vi "Send 2 PC.vi"(8 "error in (no error)":errorcluster, 10 "port":u16=5800, 11 "Camera Data In":T1 {"Camera Settings"."VideoMode" items=["640 x 480 YUY 2 30.00 fps", "640 x 480 YUY 2 20.00 fps", "640 x 480 YUY 2 15.00 fps", "640 x 480 YUY 2 10.00 fps", "640 x 480 YUY 2 7.50 fps", "1280 x 720 YUY 2 10.00 fps", "1280 x 720 YUY 2 7.50 fps", "960 x 544 YUY 2 15.00 fps", "960 x 544 YUY 2 10.00 fps", "960 x 544 YUY 2 7.50 fps", "800 x 448 YUY 2 20.00 fps", "800 x 448 YUY 2 15.00 fps", "800 x 448 YUY 2 10.00 fps", "800 x 448 YUY 2 7.50 fps", "640 x 360 YUY 2 30.00 fps", "640 x 360 YUY 2 20.00 fps", "640 x 360 YUY 2 15.00 fps", "640 x 360 YUY 2 10.00 fps", "640 x 360 YUY 2 7.50 fps", "424 x 240 YUY 2 30.00 fps", "424 x 240 YUY 2 20.00 fps", "424 x 240 YUY 2 15.00 fps", "424 x 240 YUY 2 10.00 fps", "424 x 240 YUY 2 7.50 fps", "352 x 288 YUY 2 30.00 fps", "352 x 288 YUY 2 20.00 fps", "352 x 288 YUY 2 15.00 fps", "352 x 288 YUY 2 10.00 fps", "352 x 288 YUY 2 7.50 fps", "320 x 240 YUY 2 30.00 fps", "320 x 240 YUY 2 20.00 fps", "320 x 240 YUY 2 15.00 fps", "320 x 240 YUY 2 10.00 fps", "320 x 240 YUY 2 7.50 fps", "800 x 600 YUY 2 15.00 fps", "800 x 600 YUY 2 10.00 fps", "800 x 600 YUY 2 7.50 fps", "176 x 144 YUY 2 30.00 fps", "176 x 144 YUY 2 20.00 fps", "176 x 144 YUY 2 15.00 fps", "176 x 144 YUY 2 10.00 fps", "176 x 144 YUY 2 7.50 fps", "160 x 120 YUY 2 30.00 fps", "160 x 120 YUY 2 20.00 fps", "160 x 120 YUY 2 15.00 fps", "160 x 120 YUY 2 10.00 fps", "160 x 120 YUY 2 7.50 fps", "1280 x 800 YUY 2 10.00 fps", "640 x 480 JPEG 30.00 fps", "640 x 480 JPEG 20.00 fps", "640 x 480 JPEG 15.00 fps", "640 x 480 JPEG 10.00 fps", "640 x 480 JPEG 7.50 fps", "1280 x 720 JPEG 30.00 fps", "1280 x 720 JPEG 20.00 fps", "1280 x 720 JPEG 15.00 fps", "1280 x 720 JPEG 10.00 fps", "1280 x 720 JPEG 7.50 fps", "960 x 544 JPEG 30.00 fps", "960 x 544 JPEG 20.00 fps", "960 x 544 JPEG 15.00 fps", "960 x 544 JPEG 10.00 fps", "960 x 544 JPEG 7.50 fps", "800 x 448 JPEG 30.00 fps", "800 x 448 JPEG 20.00 fps", "800 x 448 JPEG 15.00 fps", "800 x 448 JPEG 10.00 fps", "800 x 448 JPEG 7.50 fps", "640 x 360 JPEG 30.00 fps", "640 x 360 JPEG 20.00 fps", "640 x 360 JPEG 15.00 fps", "640 x 360 JPEG 10.00 fps", "640 x 360 JPEG 7.50 fps", "800 x 600 JPEG 30.00 fps", "800 x 600 JPEG 20.00 fps", "800 x 600 JPEG 15.00 fps", "800 x 600 JPEG 10.00 fps", "800 x 600 JPEG 7.50 fps", "416 x 240 JPEG 30.00 fps", "416 x 240 JPEG 20.00 fps", "416 x 240 JPEG 15.00 fps", "416 x 240 JPEG 10.00 fps", "416 x 240 JPEG 7.50 fps", "352 x 288 JPEG 30.00 fps", "352 x 288 JPEG 20.00 fps", "352 x 288 JPEG 15.00 fps", "352 x 288 JPEG 10.00 fps", "352 x 288 JPEG 7.50 fps", "176 x 144 JPEG 30.00 fps", "176 x 144 JPEG 20.00 fps", "176 x 144 JPEG 15.00 fps", "176 x 144 JPEG 10.00 fps", "176 x 144 JPEG 7.50 fps", "320 x 240 JPEG 30.00 fps", "320 x 240 JPEG 20.00 fps", "320 x 240 JPEG 15.00 fps", "320 x 240 JPEG 10.00 fps", "320 x 240 JPEG 7.50 fps", "160 x 120 JPEG 30.00 fps", "160 x 120 JPEG 20.00 fps", "160 x 120 JPEG 15.00 fps", "160 x 120 JPEG 10.00 fps", "160 x 120 JPEG 7.50 fps"]}) -> (0 "error out":errorcluster)   [LabVIEW 2015]
uses:
  Camera Data.ctl
  <vilib>/userdefined/High Color/IMAQdx.ctl
  Camera Settings.ctl
  Support Vision Code/38 Video Mode.ctl
  <vilib>/vision/driver/IMAQdx.llb/IMAQdx Buffer Number Mode.ctl
  <vilib>/vision/driver/NI_Vision_Acquisition_Software.lvlib
  <resource>/objmgr/imaqdx.rc
panel:
  out "Numeric":i32
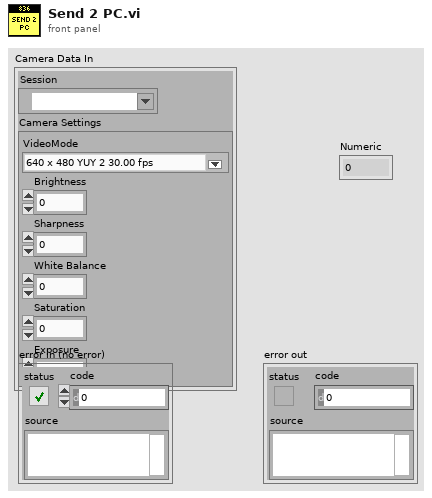
[diagram p1: front panel]
types:
  T1 = typedef "Camera Data.ctl" = cluster{"Session":T2, "Camera Settings":T3}
  T2 = typedef "IMAQdx.ctl" = refnum<k21>
  T3 = typedef "Camera Settings.ctl" = cluster{"VideoMode":T4, "Brightness":i32, "Sharpness":i32, "White Balance":i32, "Saturation":i32, "Exposure":i32}
  T4 = typedef "38 Video Mode.ctl" = u32
  T5 = typedef "NI_Vision_Acquisition_Software.lvlib/IMAQdx Buffer Number Mode.ctl" = enum32{"Next", "Last", "Buffer Number", "Every", "Last New"}
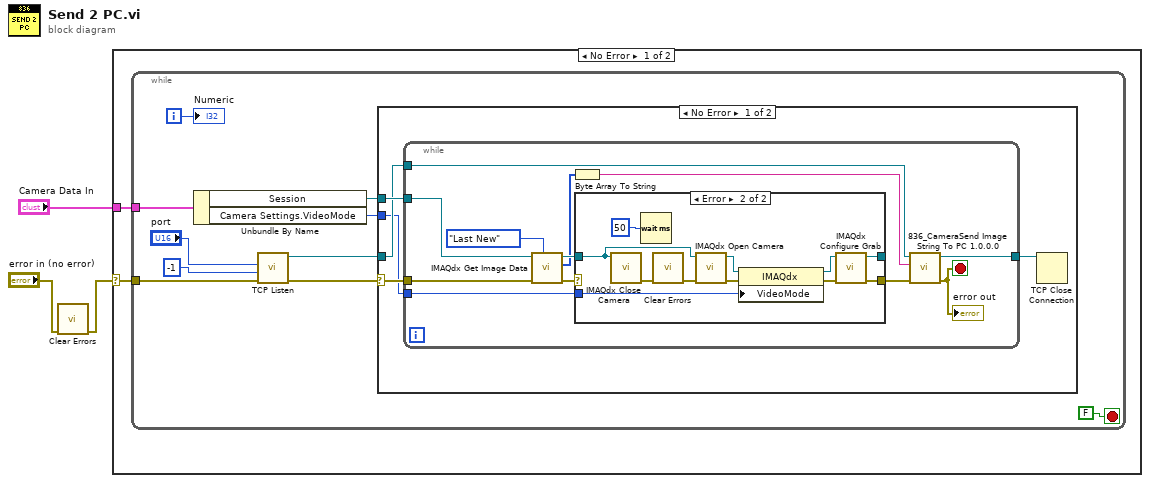
[diagram p0: block diagram]
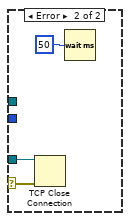
[diagram p3: hidden frame]
diagram:
  n1 = call <vilib>:"Clear Errors.vi"("error in (no error)"="error in (no error)") -> ("error out"=w1:errorcluster)  [unwired: 5 in, 1 out]
  n2 = case shown="No Error" w1 {
    selector: w1 -> [w4 _]
    tunnel: "Camera Data In" -> [w5 _]
    frame No Error {
      n3 = while {
        tunnel: w4 -> [w14]
        tunnel: w5 -> [w9]
        i -> [w6]
        stop <- FALSE stop-if-true
        n4 = Unbundle By Name(w9) -> ("Session"=w8:T2, "Camera Settings.VideoMode"=w7:T4)
        n5 = call <vilib>:"TCP Listen.vi"("error in (no error)"=w14, "timeout ms (wait forever: -1)"=-1, "port"="port") -> ("error out"=w13:errorcluster, "connection ID"=w10:refnum<k5>)  [unwired: 1 in, 6 out]
        n6 = case shown="No Error" w13 {
          selector: w13 -> [w19 w47]
          tunnel: w8 -> [w20 _]
          tunnel: w10 -> [w18 w48]
          tunnel: w7 -> [w16 _]
          frame No Error {
            n7 = while {
              tunnel: w20 -> [w31]
              tunnel: w19 -> [w25]
              tunnel: w18 -> [w24]
              tunnel: [w23] -> w17
              tunnel: w16 -> [w21]
              stop <- w22 stop-if-true
              n8 = call <vilib>:"IMAQdx Get Image Data.vi"("Buffer Number Mode (Next)"=IMAQdx_Buffer_Number_Mode."Last New", "error in"=w25, "Session In"=w31) -> ("error out"=w30:errorcluster, "Image Data Array"=w28:u8[], "Session Out"=w29:T2)  [unwired: 5 in, 1 out]
              n9 = Byte Array To String(unsigned byte array=w28) -> (string=w27:string)
              n10 = case shown="Error" w30 {
                selector: w30 -> [w33 _]
                tunnel: w29 -> [w34 w43]
                tunnel: [w33 w38] -> w26
                tunnel: [w34 w37] -> _
                tunnel: w21 -> [_ w36]
                frame No Error {
                }
                frame Error {
                  n11 = call <vilib>:"IMAQdx Close Camera.vi"("Session In"=w43) -> ("error out"=w45:errorcluster)  [unwired: 10 in]
                  n12 = Wait (ms)(milliseconds to wait=u32 50) -> ()  [unwired: 1 out]
                  n13 = call <vilib>:"Clear Errors.vi"("error in (no error)"=w45) -> ("error out"=w44:errorcluster)  [unwired: 5 in, 1 out]
                  n14 = call <vilib>:"IMAQdx Open Camera.vi"("error in"=w44, "Session In"=w43) -> ("error out"=w41:errorcluster, "Session Out"=w42:T2)  [unwired: 8 in]
                  n15 = property class="IMAQdx"(reference=w42, error in=w41, "VideoMode"=w36) -> (reference out=w40:T2, error out=w39:errorcluster)
                  n16 = call <vilib>:"IMAQdx Configure Grab.vi"("error in"=w39, "Session In"=w40) -> ("error out"=w38:errorcluster, "Session Out"=w37:T2)  [unwired: 8 in]
                }
              }
              n17 = call "836_CameraSend Image String To PC 1.0.0.0.vi"("error in (no error)"=w26, "String"=w27, "TCP Connection ID"=w24) -> ("error out"=w22:errorcluster, "TCP Connection ID out"=w23:refnum<k5>)  [unwired: 7 out]
              "error out" <- w22
            }
            n18 = TCP Close Connection(connection ID=w17) -> ()  [unwired: 1 in, 3 out]
          }
          frame Error {
            n19 = TCP Close Connection(connection ID=w48, error in (no error)=w47) -> ()  [unwired: 3 out]
            n20 = Wait (ms)(milliseconds to wait=u32 50) -> ()  [unwired: 1 out]
          }
        }
        "Numeric" <- w6
      }
    }
    frame Error {
    }
  }
